vi "photometry_Bellot_2020.vi"() -> ()   [LabVIEW 2015]
panel:
  out "Waveform Chart 4":dynamicdata(graph)
  out "Waveform Chart 3":dynamicdata(graph)
  out "Waveform Chart 2":dynamicdata(graph)
  out "Waveform Chart":dynamicdata(graph)
  in  "Raw_data":path=path "test.tdms" caption="Filename"
  out "ch4 210":waveform(dbl)(graph)
  out "ch4 500":waveform(dbl)(graph)
  out "ch3 500":waveform(dbl)(graph)
  out "ch3 210":waveform(dbl)(graph)
  out "TTLs":waveform(dbl)[](graph)
  in  "Offset 2":dbl caption="Offset"
  in  "Offset":dbl
  in  "Amplitude 2":dbl=1.0 caption="Amplitude"
  in  "Amplitude":dbl=1.0
  out "LEDs":dynamicdata(graph)
  in  "stop (F) 2":bool caption="stop (F)"
  in  "Demodulated data":path=path "test.tdms" caption="Filename"
  out "ch2 210":waveform(dbl)(graph)
  out "ch2 500":waveform(dbl)(graph)
  out "ch1 500":waveform(dbl)(graph)
  out "ch1 210":waveform(dbl)(graph)
  in  "stop (F)":bool
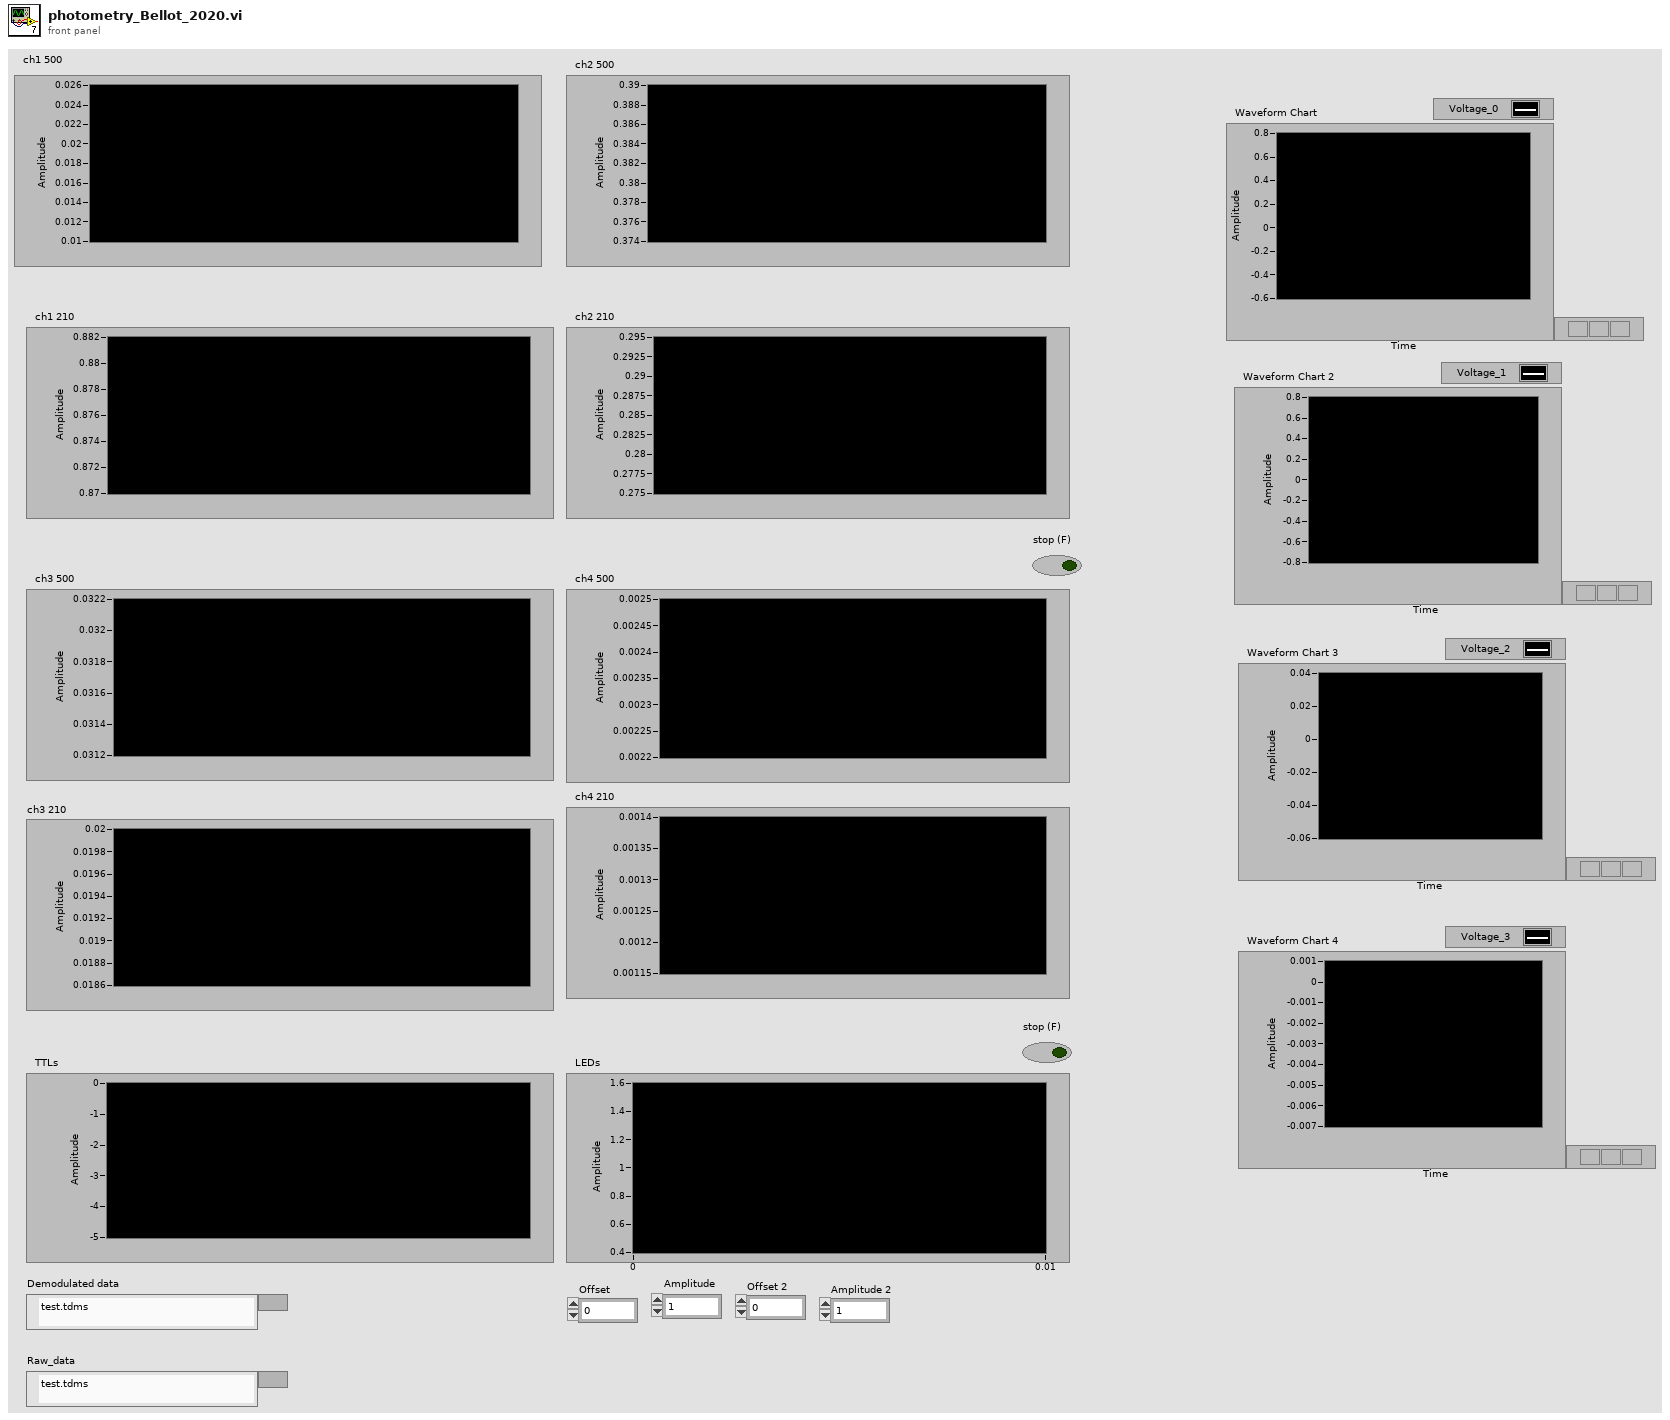
[diagram p1: front panel]
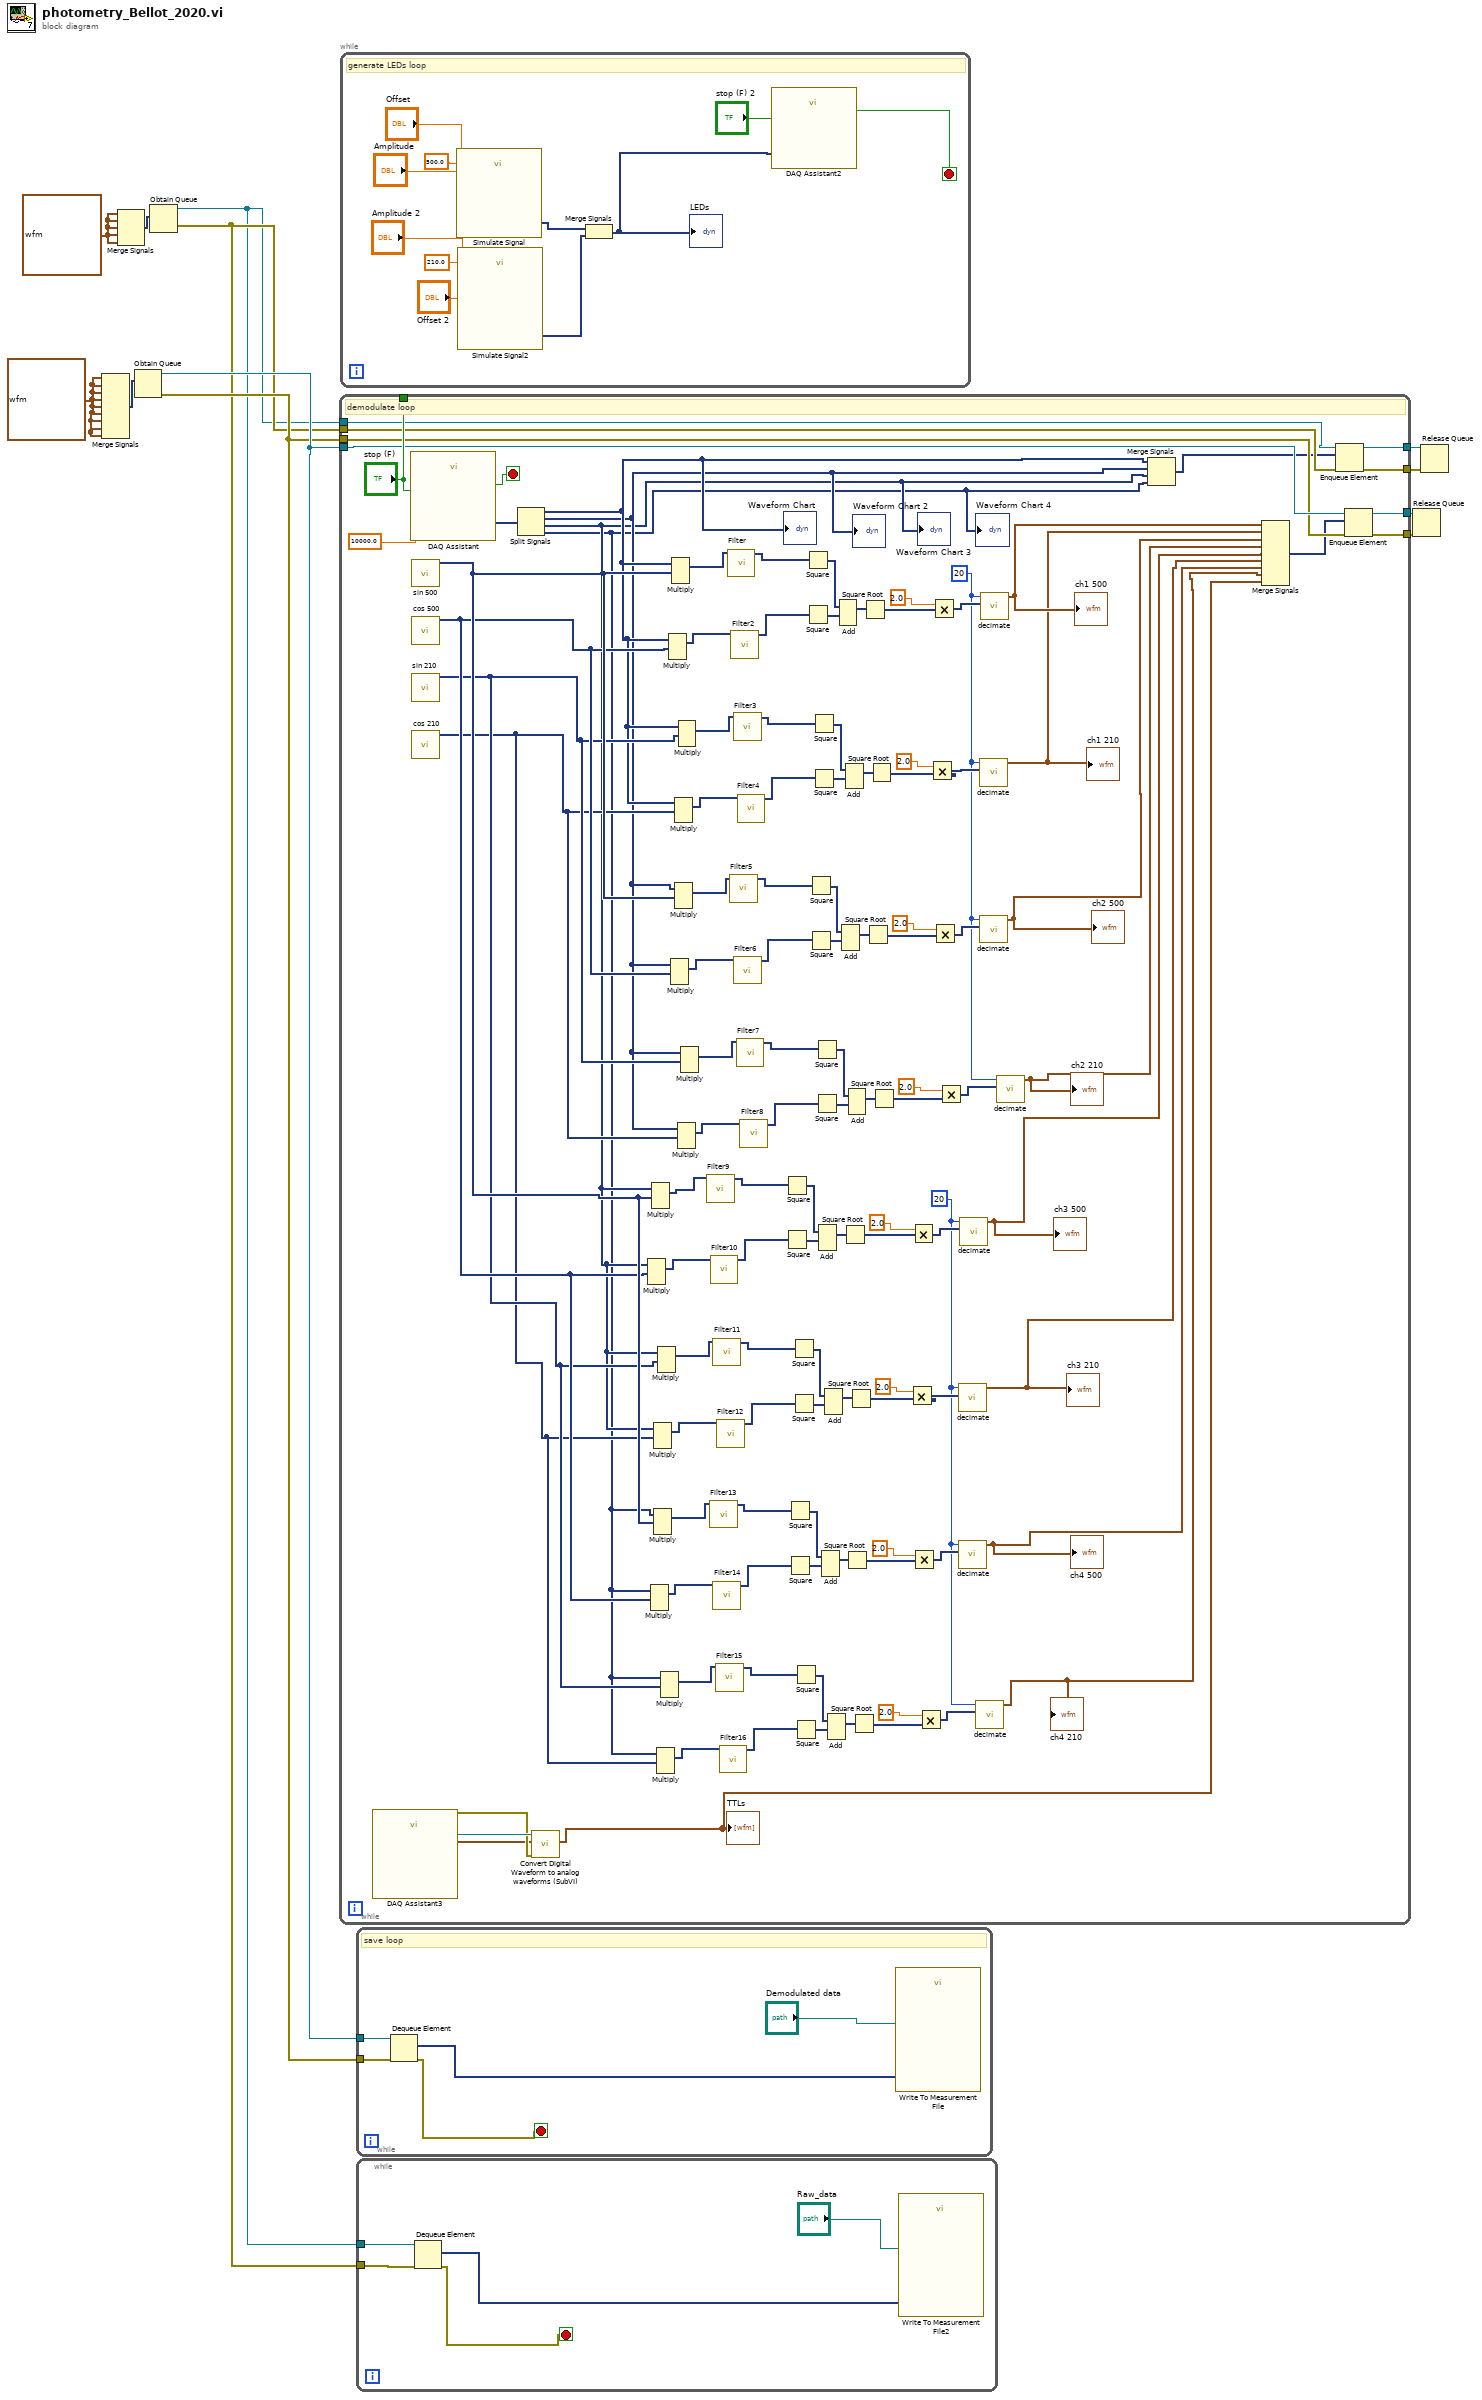
[diagram p0: block diagram]
diagram:
  w5 = waveform(dbl) {"t0"=timestamp(0 s since 1904-01-01), "dt"=1.0, "Y"=[]} ("waveform")
  w7 = waveform(dbl) {"t0"=timestamp(0 s since 1904-01-01), "dt"=1.0, "Y"=[]} ("waveform")
  n1 = Merge Signals(w7, w7, w7, w7, w7, w7, w7, w7, w7) -> (w12:dynamicdata)
  n2 = Merge Signals(w5, w5, w5, w5, w5) -> (w6:dynamicdata)
  n3 = Obtain Queue(element data type=w12) -> (queue out=w9:refnum<queue>, error out=w8:errorcluster)  [unwired: 4 in, 1 out]
  n4 = Obtain Queue(element data type=w6) -> (queue out=w1:refnum<queue>, error out=w2:errorcluster)  [unwired: 4 in, 1 out]
  n5 = while {
    tunnel: ["stop (F)"] -> _
    tunnel: [w88] -> w11
    tunnel: [w87] -> w10
    tunnel: w9 -> [w86]
    tunnel: w8 -> [w85]
    tunnel: w1 -> [w22]
    tunnel: w2 -> [w21]
    tunnel: [w20] -> w4
    tunnel: [w19] -> w3
    stop <- w128 stop-if-true
    w39 = 20 ("Divide by")
    w78 = 20 ("Divide by")
    # "demodulate loop"
    n6 = call "DAQ Assistant3"() -> ("task out"=w84:refnum<k21>, "data"=w18:digitalwaveform[], "error out"=w83:errorcluster)  [unwired: 16 in, 1 out]
    n7 = call "DAQ Assistant"("rate"=10000.0, "stop (F)"="stop (F)") -> ("data"=w127:dynamicdata, "stopped"=w128:bool)  [unwired: 14 in, 2 out]
    n8 = call "sin 500"() -> ("Sine"=w38:dynamicdata)  [unwired: 14 in, 1 out]
    n9 = call "cos 500"() -> ("Sine"=w37:dynamicdata)  [unwired: 14 in, 1 out]
    n10 = call "sin 210"() -> ("Sine"=w36:dynamicdata)  [unwired: 14 in, 1 out]
    n11 = call "cos 210"() -> ("Sine"=w35:dynamicdata)  [unwired: 14 in, 1 out]
    n12 = Split Signals(w127) -> (w16:dynamicdata, w15:dynamicdata, w14:dynamicdata, w13:dynamicdata)  [unwired: 4 in]
    "Waveform Chart" <- w16
    "Waveform Chart 2" <- w15
    "Waveform Chart 3" <- w14
    "Waveform Chart 4" <- w13
    n13 = call "Convert Digital Waveform to analog waveforms (SubVI).vi"("error in (no error)"=w83, "Digital waveform in"=w18, "Refnum in"=w84) -> ("Analog waveform array out"=w25:waveform(dbl)[])  [unwired: 6 in, 2 out]
    "TTLs" <- w25
    n14 = Multiply(1:w37, 2:w14) -> (0:w71:dynamicdata)  [unwired: 1 in, 1 out]
    n15 = Multiply(1:w37, 2:w13) -> (0:w55:dynamicdata)  [unwired: 1 in, 1 out]
    n16 = Multiply(1:w38, 2:w14) -> (0:w24:dynamicdata)  [unwired: 1 in, 1 out]
    n17 = Multiply(1:w35, 2:w14) -> (0:w64:dynamicdata)  [unwired: 1 in, 1 out]
    n18 = Multiply(1:w38, 2:w13) -> (0:w53:dynamicdata)  [unwired: 1 in, 1 out]
    n19 = Multiply(1:w35, 2:w13) -> (0:w46:dynamicdata)  [unwired: 1 in, 1 out]
    n20 = Multiply(1:w36, 2:w14) -> (0:w62:dynamicdata)  [unwired: 1 in, 1 out]
    n21 = Multiply(1:w36, 2:w13) -> (0:w44:dynamicdata)  [unwired: 1 in, 1 out]
    n22 = Multiply(1:w37, 2:w16) -> (0:w120:dynamicdata)  [unwired: 1 in, 1 out]
    n23 = Multiply(1:w37, 2:w15) -> (0:w102:dynamicdata)  [unwired: 1 in, 1 out]
    n24 = Multiply(1:w38, 2:w16) -> (0:w118:dynamicdata)  [unwired: 1 in, 1 out]
    n25 = Multiply(1:w35, 2:w16) -> (0:w111:dynamicdata)  [unwired: 1 in, 1 out]
    n26 = Multiply(1:w38, 2:w15) -> (0:w100:dynamicdata)  [unwired: 1 in, 1 out]
    n27 = Multiply(1:w35, 2:w15) -> (0:w93:dynamicdata)  [unwired: 1 in, 1 out]
    n28 = Multiply(1:w36, 2:w16) -> (0:w109:dynamicdata)  [unwired: 1 in, 1 out]
    n29 = Multiply(1:w36, 2:w15) -> (0:w91:dynamicdata)  [unwired: 1 in, 1 out]
    n30 = call "Filter9"("Signal"=w24) -> ("Filtered Signal"=w23:dynamicdata)  [unwired: 9 in, 1 out]
    n31 = call "Filter13"("Signal"=w53) -> ("Filtered Signal"=w54:dynamicdata)  [unwired: 9 in, 1 out]
    n32 = call "Filter10"("Signal"=w71) -> ("Filtered Signal"=w72:dynamicdata)  [unwired: 9 in, 1 out]
    n33 = call "Filter11"("Signal"=w62) -> ("Filtered Signal"=w63:dynamicdata)  [unwired: 9 in, 1 out]
    n34 = call "Filter14"("Signal"=w55) -> ("Filtered Signal"=w56:dynamicdata)  [unwired: 9 in, 1 out]
    n35 = call "Filter15"("Signal"=w44) -> ("Filtered Signal"=w45:dynamicdata)  [unwired: 9 in, 1 out]
    n36 = call "Filter12"("Signal"=w64) -> ("Filtered Signal"=w65:dynamicdata)  [unwired: 9 in, 1 out]
    n37 = call "Filter16"("Signal"=w46) -> ("Filtered Signal"=w47:dynamicdata)  [unwired: 9 in, 1 out]
    n38 = call "Filter"("Signal"=w118) -> ("Filtered Signal"=w119:dynamicdata)  [unwired: 9 in, 1 out]
    n39 = call "Filter5"("Signal"=w100) -> ("Filtered Signal"=w101:dynamicdata)  [unwired: 9 in, 1 out]
    n40 = call "Filter2"("Signal"=w120) -> ("Filtered Signal"=w121:dynamicdata)  [unwired: 9 in, 1 out]
    n41 = call "Filter3"("Signal"=w109) -> ("Filtered Signal"=w110:dynamicdata)  [unwired: 9 in, 1 out]
    n42 = call "Filter6"("Signal"=w102) -> ("Filtered Signal"=w103:dynamicdata)  [unwired: 9 in, 1 out]
    n43 = call "Filter7"("Signal"=w91) -> ("Filtered Signal"=w92:dynamicdata)  [unwired: 9 in, 1 out]
    n44 = call "Filter4"("Signal"=w111) -> ("Filtered Signal"=w112:dynamicdata)  [unwired: 9 in, 1 out]
    n45 = call "Filter8"("Signal"=w93) -> ("Filtered Signal"=w94:dynamicdata)  [unwired: 9 in, 1 out]
    n46 = Square(x=w23) -> (x^2=w74:dynamicdata)
    n47 = Square(x=w72) -> (x^2=w75:dynamicdata)
    n48 = Square(x=w54) -> (x^2=w58:dynamicdata)
    n49 = Square(x=w56) -> (x^2=w59:dynamicdata)
    n50 = Square(x=w63) -> (x^2=w67:dynamicdata)
    n51 = Square(x=w65) -> (x^2=w68:dynamicdata)
    n52 = Square(x=w45) -> (x^2=w49:dynamicdata)
    n53 = Square(x=w47) -> (x^2=w50:dynamicdata)
    n54 = Square(x=w119) -> (x^2=w123:dynamicdata)
    n55 = Square(x=w121) -> (x^2=w124:dynamicdata)
    n56 = Square(x=w101) -> (x^2=w105:dynamicdata)
    n57 = Square(x=w103) -> (x^2=w106:dynamicdata)
    n58 = Square(x=w110) -> (x^2=w114:dynamicdata)
    n59 = Square(x=w112) -> (x^2=w115:dynamicdata)
    n60 = Square(x=w92) -> (x^2=w96:dynamicdata)
    n61 = Square(x=w94) -> (x^2=w97:dynamicdata)
    n62 = Add(1:w75, 2:w74) -> (0:w73:dynamicdata)  [unwired: 1 in, 1 out]
    n63 = Add(1:w59, 2:w58) -> (0:w57:dynamicdata)  [unwired: 1 in, 1 out]
    n64 = Add(1:w68, 2:w67) -> (0:w66:dynamicdata)  [unwired: 1 in, 1 out]
    n65 = Add(1:w50, 2:w49) -> (0:w48:dynamicdata)  [unwired: 1 in, 1 out]
    n66 = Add(1:w124, 2:w123) -> (0:w122:dynamicdata)  [unwired: 1 in, 1 out]
    n67 = Add(1:w106, 2:w105) -> (0:w104:dynamicdata)  [unwired: 1 in, 1 out]
    n68 = Add(1:w115, 2:w114) -> (0:w113:dynamicdata)  [unwired: 1 in, 1 out]
    n69 = Square Root(x=w73) -> (sqrt(x)=w76:dynamicdata)
    n70 = Add(1:w97, 2:w96) -> (0:w95:dynamicdata)  [unwired: 1 in, 1 out]
    n71 = Square Root(x=w57) -> (sqrt(x)=w60:dynamicdata)
    n72 = Square Root(x=w66) -> (sqrt(x)=w69:dynamicdata)
    n73 = Square Root(x=w48) -> (sqrt(x)=w51:dynamicdata)
    n74 = Square Root(x=w122) -> (sqrt(x)=w125:dynamicdata)
    n75 = Square Root(x=w104) -> (sqrt(x)=w107:dynamicdata)
    n76 = Square Root(x=w113) -> (sqrt(x)=w116:dynamicdata)
    n77 = Square Root(x=w95) -> (sqrt(x)=w98:dynamicdata)
    n78 = Multiply(x=2.0, y=w69) -> (x*y=w42:dynamicdata)
    n79 = Multiply(x=2.0, y=w76) -> (x*y=w43:dynamicdata)
    n80 = Multiply(x=2.0, y=w60) -> (x*y=w41:dynamicdata)
    n81 = Multiply(x=2.0, y=w51) -> (x*y=w40:dynamicdata)
    n82 = Multiply(x=2.0, y=w116) -> (x*y=w81:dynamicdata)
    n83 = Multiply(x=2.0, y=w125) -> (x*y=w82:dynamicdata)
    n84 = Multiply(x=2.0, y=w107) -> (x*y=w80:dynamicdata)
    n85 = Multiply(x=2.0, y=w98) -> (x*y=w79:dynamicdata)
    n86 = call "decimate.vi"("Waveform"=w42, "Divide by"=w39) -> ("output waveform"=w28:waveform(dbl))  [unwired: 9 in]
    "ch3 210" <- w28
    n87 = call "decimate.vi"("Waveform"=w41, "Divide by"=w39) -> ("output waveform"=w27:waveform(dbl))  [unwired: 9 in]
    "ch4 500" <- w27
    n88 = call "decimate.vi"("Waveform"=w43, "Divide by"=w39) -> ("output waveform"=w29:waveform(dbl))  [unwired: 9 in]
    "ch3 500" <- w29
    n89 = call "decimate.vi"("Waveform"=w40, "Divide by"=w39) -> ("output waveform"=w26:waveform(dbl))  [unwired: 9 in]
    "ch4 210" <- w26
    n90 = call "decimate.vi"("Waveform"=w81, "Divide by"=w78) -> ("output waveform"=w32:waveform(dbl))  [unwired: 9 in]
    "ch1 210" <- w32
    n91 = call "decimate.vi"("Waveform"=w80, "Divide by"=w78) -> ("output waveform"=w31:waveform(dbl))  [unwired: 9 in]
    "ch2 500" <- w31
    n92 = call "decimate.vi"("Waveform"=w82, "Divide by"=w78) -> ("output waveform"=w33:waveform(dbl))  [unwired: 9 in]
    "ch1 500" <- w33
    n93 = call "decimate.vi"("Waveform"=w79, "Divide by"=w78) -> ("output waveform"=w30:waveform(dbl))  [unwired: 9 in]
    "ch2 210" <- w30
    n94 = Merge Signals(w16, w15, w14, w13) -> (w17:dynamicdata)
    n95 = Merge Signals(w33, w32, w31, w30, w29, w28, w27, w26, w25) -> (w34:dynamicdata)
    n96 = Enqueue Element(queue=w22, element=w17, error in (no error)=w21) -> (queue out=w20:refnum<queue>, error out=w19:errorcluster)  [unwired: 1 in, 1 out]
    n97 = Enqueue Element(queue=w86, element=w34, error in (no error)=w85) -> (queue out=w87:refnum<queue>, error out=w88:errorcluster)  [unwired: 1 in, 1 out]
  }
  n98 = while {
    stop <- w138 stop-if-true
    # "generate LEDs loop"
    n99 = call "Simulate Signal"("Offset"="Offset", "Frequency"=500.0, "Amplitude"="Amplitude") -> ("Sine"=w137:dynamicdata)  [unwired: 11 in, 1 out]
    n100 = call "Simulate Signal2"("Offset"="Offset 2", "Frequency"=210.0, "Amplitude"="Amplitude 2") -> ("Sine"=w136:dynamicdata)  [unwired: 11 in, 1 out]
    n101 = Merge Signals(w137, w136) -> (w129:dynamicdata)
    "LEDs" <- w129
    n102 = call "DAQ Assistant2"("data"=w129, "stop (F)"="stop (F) 2") -> ("stopped"=w138:bool)  [unwired: 15 in, 2 out]
  }
  n103 = while {
    tunnel: w9 -> [w143]
    tunnel: w8 -> [w142]
    stop <- w141 stop-if-true
    # "save loop"
    n104 = Dequeue Element(queue=w143, error in (no error)=w142) -> (element=w144:dynamicdata, error out=w141:errorcluster)  [unwired: 1 in, 2 out]
    n105 = call "Write To Measurement File"("Signals"=w144, "Filename"="Demodulated data") -> ()  [unwired: 15 in, 3 out]
  }
  n106 = while {
    tunnel: w1 -> [w146]
    tunnel: w2 -> [w145]
    stop <- w147 stop-if-true
    n107 = Dequeue Element(queue=w146, error in (no error)=w145) -> (element=w149:dynamicdata, error out=w147:errorcluster)  [unwired: 1 in, 2 out]
    n108 = call "Write To Measurement File2"("Signals"=w149, "Filename"="Raw_data") -> ()  [unwired: 15 in, 3 out]
  }
  n109 = Release Queue(queue=w10, error in (no error)=w11) -> ()  [unwired: 1 in, 3 out]
  n110 = Release Queue(queue=w4, error in (no error)=w3) -> ()  [unwired: 1 in, 3 out]
